vi "act-0011-1-cor.vi"() -> ()   [LabVIEW 2010]
panel:
  out "Graphe déroulant":dbl(graph)
  in  "Nombre d'itérations":i32
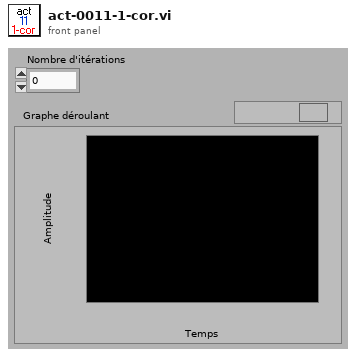
[diagram p1: front panel]
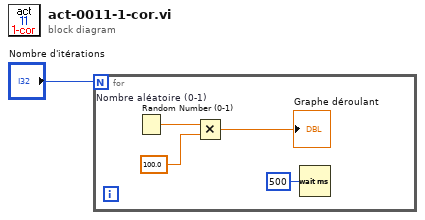
[diagram p0: block diagram]
diagram:
  n1 = for {
    N: "Nombre d'itérations" -> [_]
    n2 = Random Number (0-1) "Nombre aléatoire (0-1)"() -> (number: 0 to 1=w5:dbl)
    n3 = Multiply(x=w5, y=100.0) -> (x*y=→"Graphe déroulant":dbl)
    n4 = Wait (ms)(milliseconds to wait=u32 500 ("attente (ms)")) -> ()  [unwired: 1 out]
  }
